vi "Basic Test.vi"(11 "Data In":i32) -> (3 "Data Out":i32)   [LabVIEW 2018]
uses:
  Core/Assert API Components/Assert API Components.lvlib
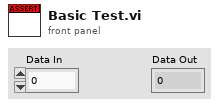
[diagram p1: front panel]
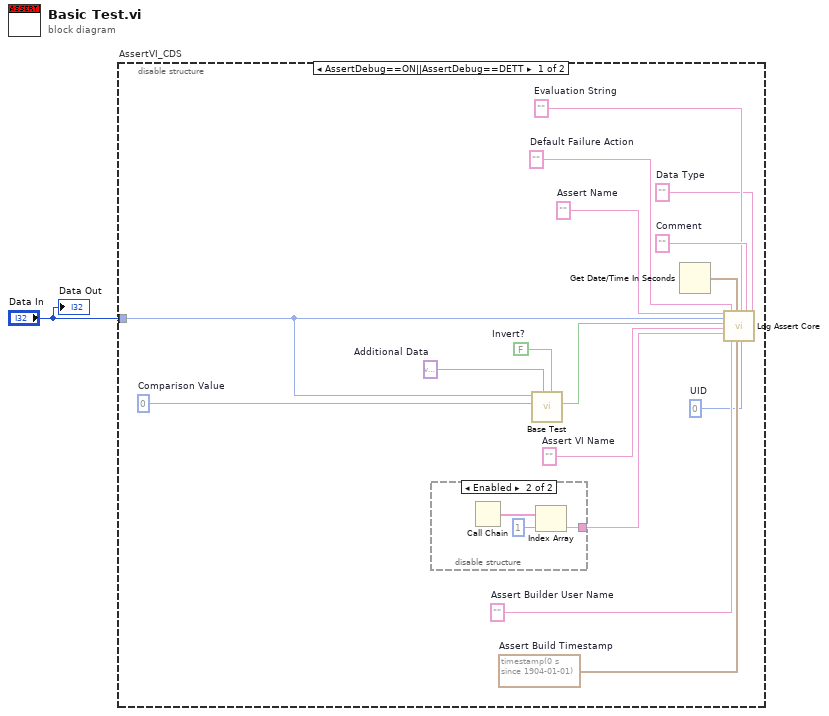
[diagram p0: block diagram]
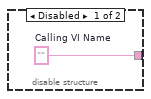
[diagram p2: hidden frame]
diagram:
  n1 = disable-structure "AssertVI_CDS" shown="AssertDebug==ON||AssertDebug==DETT" {
    disable-tunnel: "Data In" -> [w4 _]
    frame condition #0 {
      w2 = variant  # Additional Data
      w3 = FALSE  # Invert?
      w6 = 0  # UID
      w8 = ""  # Assert VI Name
      w9 = timestamp(0 s since 1904-01-01)  # Assert Build Timestamp
      w10 = ""  # Assert Builder User Name
      w11 = ""  # Data Type
      w14 = ""  # Comment
      w12 = ""  # Evaluation String
      w16 = ""  # Default Failure Action
      w17 = ""  # Assert Name
      w15 = 0  # Comparison Value
      n2 = disable-structure shown="Enabled" {
        disable-tunnel: [w18 w19] -> w5
        frame Disabled {
          w18 = ""  # Calling VI Name
        }
        frame Enabled {
          n3 = Call Chain() -> (call chain=w20:string[])
          n4 = Index Array(array=w20, index=1) -> (element=w19:string)
        }
      }
      n5 = call "Base Test.vi"("Invert?"=w3, "Additional Data"=w2, "y"=w15, "x"=w4) -> ("Equal?"=w13:bool)  [unwired: 7 in]
      n6 = Get Date/Time In Seconds() -> (seconds since 1Jan1904=w7:timestamp)
      n7 = call "Log Assert Core.vi"("Assert Name"=w17, "Data Value"=w4, "Status"=w13, "Assert VI Name"=w8, "Calling VI Name"=w5, "Failure Action"=w16, "Assert Builder User Name"=w10, "Last Update"=w7, "Assert Build Timestamp"=w9, "Evaluation String"=w12, "Assert VI UID"=w6, "Comment"=w14, "Data Type"=w11) -> ()  [unwired: 7 in]
    }
    frame condition #1 (active) {
    }
  }
  "Data Out" <- "Data In"
